vi "IMAQdx Get Camera Status.vi"(8 "error in":errorcluster, 11 "Session In":T1) -> (0 "error out":errorcluster, 2 "Destination Mode":u32(ring) items=["Unicast", "Broadcast", "Multicast"], 3 "Acquiring?":bool)   [LabVIEW 2020, in "NI_Vision_Acquisition_Software.lvlib"]
doc: "Get current status of camera."
uses:
  NI_Vision_Acquisition_Software.lvlib
  IMAQdx.ctl
  niimaqdx.dll
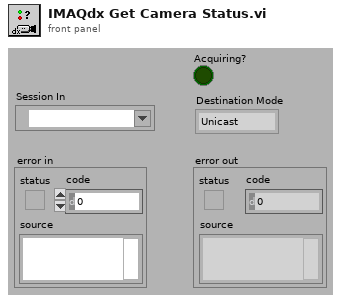
[diagram p1: front panel]
types:
  T1 = typedef "IMAQdx.ctl" = refnum<k21>
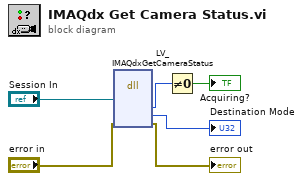
[diagram p0: block diagram]
diagram:
  n1 = dll-call lib="niimaqdx.dll" fn="LV_IMAQdxGetCameraStatus"("interfaceName"="Session In", "error in"="error in") -> ("acquiring"=w4:u32, "destinationMode"=→"Destination Mode":u32, "error in"=→"error out":errorcluster)  [unwired: 7 in, 2 out]
  n2 = Not Equal To 0?(x=w4) -> (x != 0?=→"Acquiring?":bool)
